vi "Multiply.vi"(1 "x":sgl, 2 "y":sgl, 4 "Multiplier":refnum<class "Multiplier.lvclass">) -> (6 "x*y":sgl)   [LabVIEW 2017, in "Multiplier.lvclass"]
uses:
  Multiplier.lvclass
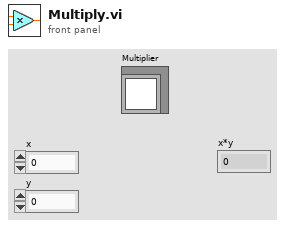
[diagram p1: front panel]
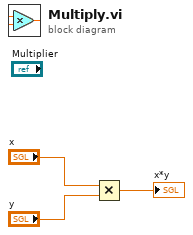
[diagram p0: block diagram]
diagram:
  n1 = Multiply(x="x", y="y") -> (x*y=→"x*y":sgl)
